vi "Weather Monitor.vi"() -> ()   [LabVIEW 2023]
doc: "The main VI for the Weather Monitor Client built application. This VI uses the HTTP client to call the Weather Monitor web service, which can be hosted in the Weather Monitor Simulator built application or debugged inside of the project."
uses:
  Weather Monitor Views.lvlib
  support/Message Queue/Weather Message Queue.lvlib
  Weather Request Loop.lvlib
  Weather Wait Loop.lvlib
panel:
  in  "Close Button":bool
  in  "Start Button":bool
  in  "Display format":u16(ring) items=["Graph", "Table", "Raw Values"]
  in  "Refresh rate":i32=2000 caption="Refresh rate [ms]" step=100
  in  "Port":u16=80 step=1
  in  "Remote host/IP address":string="127.0.0.1"
  # "Overview: Demonstrates the use of the HTTP Client to call the Weather Monitor web service hosted by the Weather Simulator application.\nRequirements: LabVIEW Full Development System\nInstructions:\n1. Build and run the Weather Simulator (server) build specification.\n2. Run this vi or build and run the Weather Monitor (client) build specification.\n3. Select a display format and click the Start button below.\n4. See README.htm for more information, including how to run the web service for debugging."
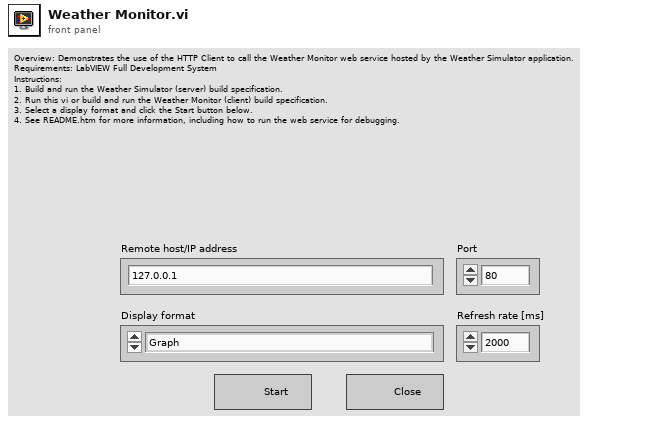
[diagram p1: front panel]
types:
  T1 = typedef "Weather Message Queue.lvlib/All Message Queues.ctl" = cluster{"View":refnum<queue>, "Request":refnum<queue>, "Wait":refnum<queue>}
  T2 = enum32{"invalid app kind", "Development System", "Run Time System", "Student Edition", "Embedded LabVIEW", "Evaluation", "Custom"}
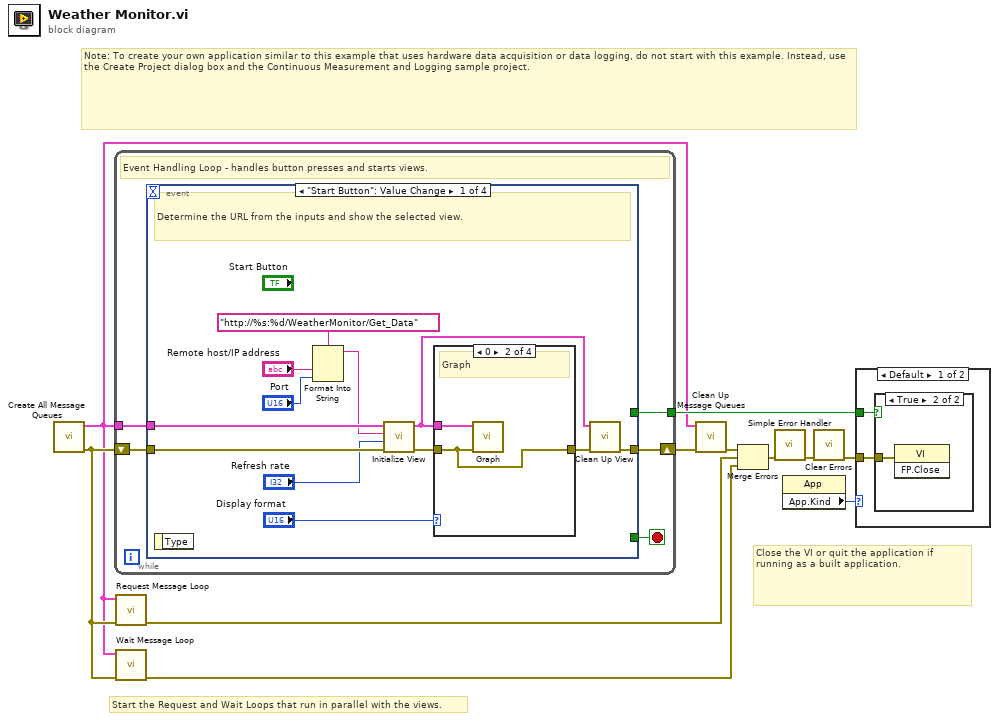
[diagram p0: block diagram]
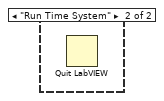
[diagram p3: hidden frame]
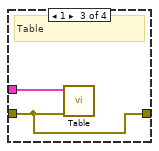
[diagram p5: hidden frame]
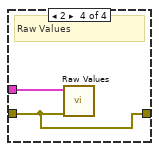
[diagram p6: hidden frame]
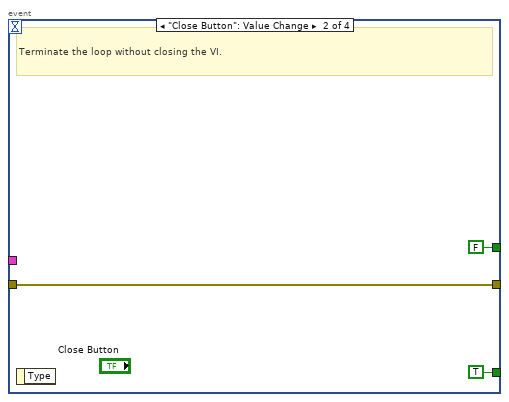
[diagram p7: hidden frame]
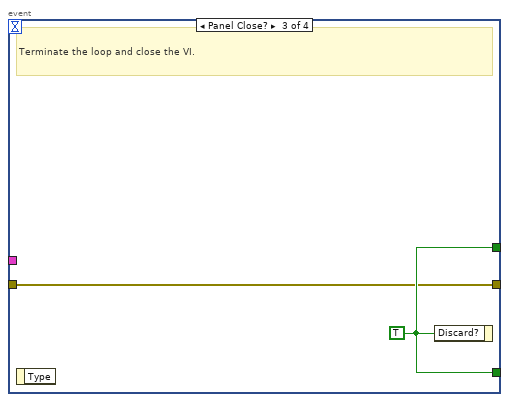
[diagram p8: hidden frame]
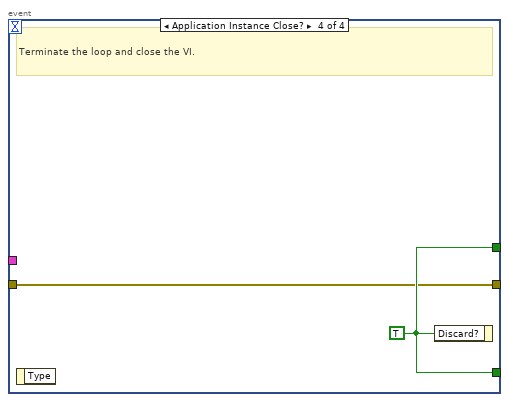
[diagram p9: hidden frame]
diagram:
  # "Start the Request and Wait Loops that run in parallel with the views."
  # "Note: To create your own application similar to this example that uses hardware data acquisition or data logging, do not start with this example. Instead, use the Create Project dialog box and the Continuous Measurement and Logging sample project."
  # "Close the VI or quit the application if running as a built application."
  n1 = call "Create All Message Queues.vi"() -> ("error out"=w9:errorcluster, "Message Queues out"=w1:T1)  [unwired: 10 in]
  n2 = while {
    tunnel: [w15] -> w11
    tunnel: w1 -> [w12]
    shift-right: [w13] -> w8
    shift-left: w9 -> [w14]
    stop <- w16 stop-if-true
    # "Event Handling Loop - handles button presses and starts views."
    n3 = event shown="[0] \"Start Button\": Value Change" {
      selector: _ -> [_ _ _ _]
      dyn-events: _ -> [_ _ _ _]
      timeout: _ -> [_ _ _ _]
      tunnel: [_ TRUE ("Cancel Button") w40 w42] -> w16
      tunnel: [_ FALSE ("Discard?") w40 w42] -> w15
      tunnel: w14 -> [w26 w36 w39 w41]
      tunnel: [w18 w36 w39 w41] -> w13
      tunnel: w12 -> [w22 _ _ _]
      event "Start Button": Value Change {
        # "Determine the URL from the inputs and show the selected view."
        n4 = event-data() -> ()  [unwired: 1 in, 1 out]
        n5 = Format Into String(format string="http://%s:%d/WeatherMonitor/Get_Data", "Remote host/IP address", "Port") -> (resulting string=w21:string)  [unwired: 2 in, 1 out]
        n6 = call "Initialize View.vi"("error in (no error)"=w26, "Refresh rate"="Refresh rate", "URL"=w21, "Message Queues in"=w22) -> ("error out"=w27:errorcluster, "dup Message Queues"=w17:T1)  [unwired: 6 in]
        n7 = case shown="0" "Display format" {
          tunnel: w17 -> [_ w31 w33 w35]
          tunnel: w27 -> [w29 w30 w32 w34]
          tunnel: [w29 w30 w32 w34] -> w19
          frame Default {
          }
          frame 0 {
            # "Graph"
            n8 = call "Graph.vi"("error in (no error)"=w30, "Message Queues"=w31) -> ()  [unwired: 10 in]
          }
          frame 1 {
            # "Table"
            n9 = call "Table.vi"("Error In"=w32, "Message Queues"=w33) -> ()  [unwired: 10 in]
          }
          frame 2 {
            # "Raw Values"
            n10 = call "Raw Values.vi"("error in (no error)"=w34, "Message Queues"=w35) -> ()  [unwired: 10 in]
          }
        }
        n11 = call "Clean Up View.vi"("error in (no error)"=w19, "Message Queues in"=w17) -> ("error out"=w18:errorcluster)  [unwired: 8 in, 1 out]
      }
      event "Close Button": Value Change {
        # "Terminate the loop without closing the VI."
        n12 = event-data() -> ()  [unwired: 1 in, 1 out]
      }
      event Panel Close? {
        w40 = TRUE ("Discard?")
        # "Terminate the loop and close the VI."
        n13 = event-data() -> ()  [unwired: 1 in, 1 out]
        n14 = event-data("Discard?"=w40) -> ()  [unwired: 1 in, 1 out]
      }
      event Application Instance Close? {
        w42 = TRUE ("Discard?")
        # "Terminate the loop and close the VI."
        n15 = event-data() -> ()  [unwired: 1 in, 1 out]
        n16 = event-data("Discard?"=w42) -> ()  [unwired: 1 in, 1 out]
      }
    }
  }
  n17 = call "Request Message Loop.vi"("error in (no error)"=w9, "Message Queues"=w1) -> ("error out"=w7:errorcluster)  [unwired: 9 in]
  n18 = call "Wait Message Loop.vi"("error in (no error)"=w9, "Message Queues"=w1) -> ("error out"=w6:errorcluster)  [unwired: 9 in]
  n19 = call "Clean Up Message Queues.vi"("error in (no error)"=w8, "Message Queues"=w1) -> ("error out"=w2:errorcluster)  [unwired: 9 in]
  n20 = Merge Errors(w2, w7, w6) -> (w5:errorcluster)
  n21 = call <vilib>:"Simple Error Handler.vi"("error in (no error)"=w5) -> ("error out"=w3:errorcluster)  [unwired: 4 in, 4 out]
  n22 = property class="App"() -> ("App.Kind"=w10:T2)  [unwired: 2 in, 2 out]
  n23 = call <vilib>:"Clear Errors.vi"("error in (no error)"=w3) -> ("error out"=w4:errorcluster)  [unwired: 5 in, 1 out]
  n24 = case shown="Default" w10 {
    tunnel: w11 -> [w44 _]
    tunnel: w4 -> [w43 _]
    frame Default {
      n25 = case shown="True" w44 {
        tunnel: w43 -> [_ w45]
        frame False {
        }
        frame True {
          n26 = invoke class="VI" method="FP.Close"(error in=w45) -> ()  [unwired: 2 in, 3 out]
        }
      }
    }
    frame "Run Time System" {
      n27 = Quit LabVIEW() -> ()  [unwired: 1 in]
    }
  }
